vi "PH_DIM.add Double Service.vi"(0 "i ref in":refnum<vi>, 1 "Service Name":string="N/A", 2 "Double Value":dbl, 5 "error in (no error)":errorcluster) -> (14 "i ref out":refnum<vi>, 17 "Service ID":i32, 19 "error out":errorcluster)   [LabVIEW 2014, in "PH_Common.lvlib"]
doc: "This VI publishes a double number opening a service \"<instancename>_ServiceName\", if no error comes in, and the ServiceName is not N/A. For further use, the Service ID is given out (it is \"-1\" if the service has not been added)."
uses:
  PH_Common.lvlib
  lib.lib/DimLVEvent/LVDimInterface/LVDimInterface.lvlib
  CSCore/CSSystem/CSSystemLib/CSSystemLib.lvlib
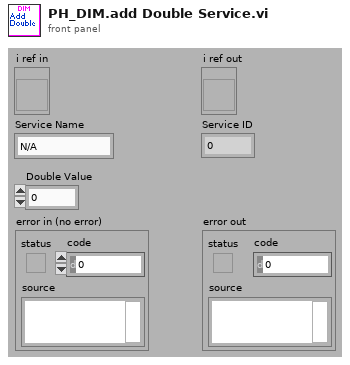
[diagram p1: front panel]
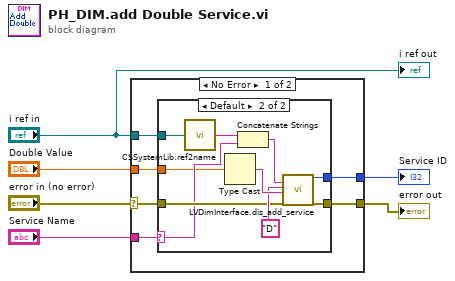
[diagram p0: block diagram]
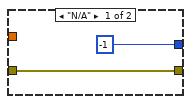
[diagram p2: hidden frame]
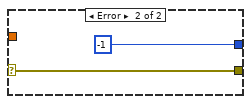
[diagram p3: hidden frame]
diagram:
  n1 = case shown="No Error" "error in (no error)" {
    selector: "error in (no error)" -> [w9 w26]
    tunnel: [w12 -1 ("my_serviceID")] -> w6
    tunnel: [w11 w26] -> w5
    tunnel: "Double Value" -> [w8 _]
    tunnel: "i ref in" -> [w10 _]
    tunnel: "Service Name" -> [w7 _]
    frame No Error {
      n2 = case shown="Default" w7 {
        selector: w7 -> [_ w17]
        tunnel: [-1 ("my_serviceID") w16] -> w12
        tunnel: [w14 w18] -> w11
        tunnel: w10 -> [_ w20]
        tunnel: w9 -> [w14 w19]
        tunnel: w8 -> [_ w15]
        frame "N/A" {
        }
        frame Default {
          n3 = call "CSSystemLib.ref2name.vi"("obj refnum"=w20) -> ("name"=w22:string)
          n4 = Type Cast(x=w15) -> (*(type *) &x=w24:string)  [unwired: 1 in]
          n5 = Concatenate Strings(w22, w17) -> (w21:string)
          n6 = call "LVDimInterface.dis_add_service.vi"("serviceName"=w21, "typeDescriptor"="D", "data"=w24, "error in (no error)"=w19) -> ("my_serviceID"=w16:i32, "error out"=w18:errorcluster)  [unwired: 14 in]
        }
      }
    }
    frame Error {
    }
  }
  "Service ID" <- w6
  "error out" <- w5
  "i ref out" <- "i ref in"
